vi "Update Global References.vi"(8 "error in":errorcluster) -> (0 "error out":errorcluster)   [LabVIEW 2026, in "Custom Device Test Bench.lvlib"]
uses:
  Custom Device Test Bench.lvlib
  <vilib>/NI VeriStand/Custom Device API/Data Table Ref.ctl
  <vilib>/NI VeriStand/Custom Device API/Custom Device API.lvlib
  <vilib>/NI VeriStand/Custom Device API/Global Data Refs.vi
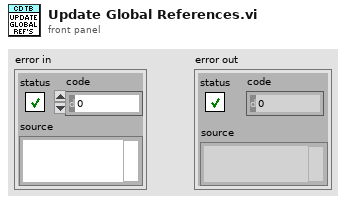
[diagram p1: front panel]
types:
  T1 = typedef "Custom Device API.lvlib/Data Table Ref.ctl" = cluster{"Ptr.Beg":u64, "Ptr.End":u64}
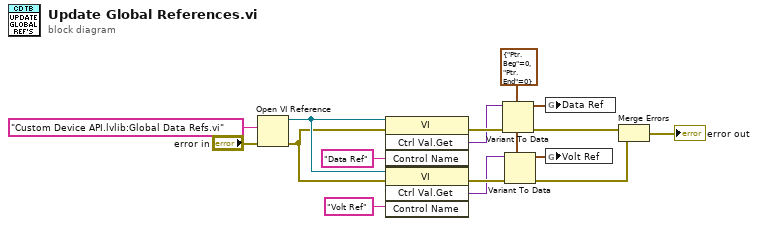
[diagram p0: block diagram]
diagram:
  w4 = T1 {"Ptr.Beg"=0, "Ptr.End"=0} ("Data Table Ref")
  n1 = Open VI Reference(vi path="Custom Device API.lvlib:Global Data Refs.vi", error in (no error)="error in") -> (vi reference=w9:refnum<vi>, error out=w1:errorcluster)  [unwired: 4 in]
  n2 = invoke class="VI" method="Ctrl Val.Get"(reference=w9, error in=w1, "Control Name"="Data Ref") -> (error out=w15:errorcluster, "Get Control Value Variant"=w5:variant)  [unwired: 1 in, 2 out]
  n3 = invoke class="VI" method="Ctrl Val.Get"(reference=w9, error in=w1, "Control Name"="Volt Ref") -> (error out=w14:errorcluster, "Get Control Value Variant"=w6:variant)  [unwired: 1 in, 2 out]
  n4 = Variant To Data(error in=w15, type=w4, Variant=w5) -> (data=w3:T1, error out=w13:errorcluster)
  n5 = Variant To Data(error in=w14, type=w4, Variant=w6) -> (data=w2:T1, error out=w12:errorcluster)
  n6 = global write "Global Data Refs.vi" "Data Ref"(w3) -> ()
  n7 = global write "Global Data Refs.vi" "Volt Ref"(w2) -> ()
  n8 = Merge Errors(w13, w12) -> (→"error out":errorcluster)
